vi "Get Meta Data.vi"(0 "Measurement Client Wrapper in":refnum<class "Measurement Client Wrapper.lvclass">, 11 "error in":errorcluster) -> (4 "Measurement Client Wrapper out":refnum<class "Measurement Client Wrapper.lvclass">, 15 "error out":errorcluster)   [LabVIEW 2020, in "Measurement Client Wrapper.lvclass"]
uses:
  Measurement Client Wrapper.lvclass
  Measurement Client Wrapper.lvclass/Measurement Client Wrapper.ctl
  Typedefs/Measurement Parameters.ctl
  Typedefs/Measurement Parameter Details.ctl
  Typedefs/Measurement DataType.ctl
  Measurement_lv_client/Measurement_lv_client Class/Measurement_lv_client.lvclass
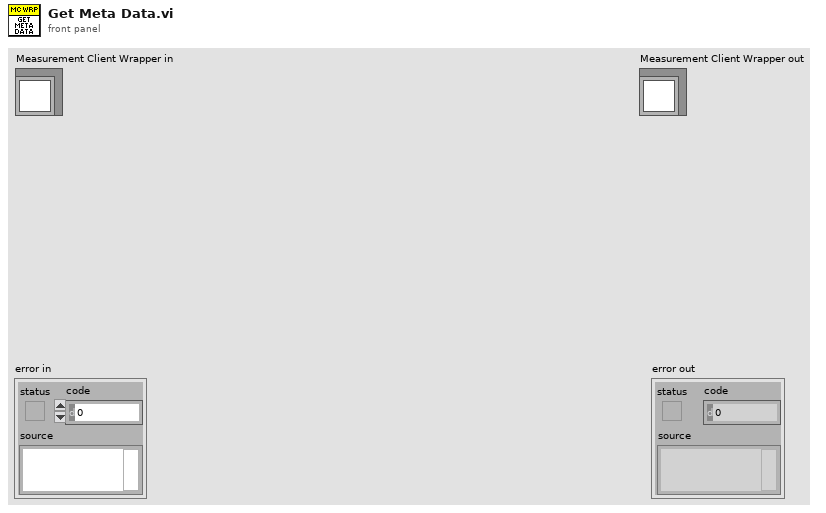
[diagram p1: front panel]
types:
  T1 = typedef "Measurement Client Wrapper.lvclass/Measurement Parameters.ctl" = cluster{"Configuration Parameters MessageType":string, "Configuration Parameter[]":T2[], "Output Parameters MessageType":string, "Output Parameter[]":T2[]}
  T2 = typedef "Measurement Client Wrapper.lvclass/Measurement Parameter Details.ctl" = cluster{"Name":string, "Parent":string, "ProtobufID":i32, "Measurement DataType":T3, "Array Dimension":i32}
  T3 = typedef "Measurement Client Wrapper.lvclass/Measurement DataType.ctl" = enum16{"UNSPECIFIED", "BOOL", "DOUBLE", "FLOAT", "INT32", "INT64", "STRING", "UINT32", "UINT64"}
  T4 = typedef "Measurement_lv_client.lvlib/Measurement_lv_client.lvclass/Measurement_v1_GetMetadataResponse_Data.ctl" = cluster{"measurement_details":T5, "measurement_parameters":T6, "user_interface_details":T9}
  T5 = typedef "Measurement_lv_client.lvlib/Measurement_lv_client.lvclass/Measurement_v1_MeasurementDetails_Data.ctl" = cluster{"display_name":string, "version":string, "measurement_type":string, "product_type":string}
  T6 = typedef "Measurement_lv_client.lvlib/Measurement_lv_client.lvclass/Measurement_v1_MeasurementParameters_Data.ctl" = cluster{"configuration_parameters_messagetype":string, "configuration_parameters":T7[], "output_parameters_messagetype":string, "output_parameters":T8[]}
  T7 = typedef "Measurement_lv_client.lvlib/Measurement_lv_client.lvclass/Measurement_v1_ConfigurationParameter_Data.ctl" = cluster{"protobuf_id":i32, "type":i32, "ArrayDimension":i32, "name":string, "parent":string}
  T8 = typedef "Measurement_lv_client.lvlib/Measurement_lv_client.lvclass/Measurement_v1_OutputParameter_Data.ctl" = cluster{"protobuf_id":i32, "type":i32, "ArrayDimension":i32, "name":string, "parent":string}
  T9 = typedef "Measurement_lv_client.lvlib/Measurement_lv_client.lvclass/Measurement_v1_UserInterfaceDetails_Data.ctl" = cluster{"configuration_ui_url":string}
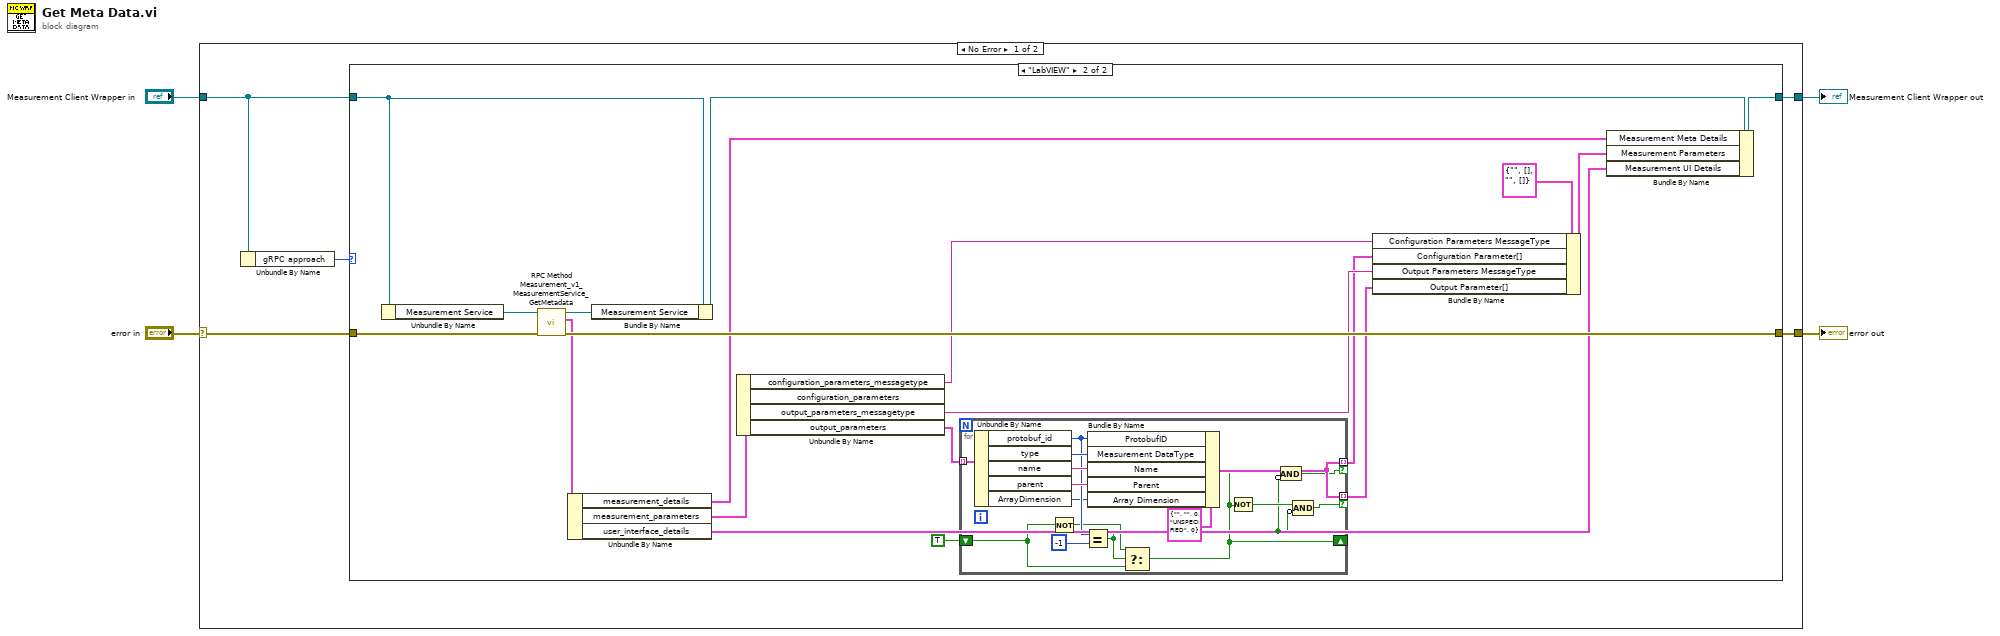
[diagram p0: block diagram]
diagram:
  n1 = case shown="No Error" "error in" {
    selector: "error in" -> [w9 w48]
    tunnel: [w7 w48] -> w3
    tunnel: [w8 w47] -> w1
    tunnel: "Measurement Client Wrapper in" -> [w6 w47]
    frame No Error {
      n2 = Unbundle By Name(w6) -> ("gRPC approach"=w5:enum16{".NET", "LabVIEW"})
      n3 = case shown="\"LabVIEW\"" w5 {
        tunnel: w9 -> [w11 w28]
        tunnel: [w10 w13] -> w8
        tunnel: [w11 w27] -> w7
        tunnel: w6 -> [w10 w30]
        frame ".NET", Default {
        }
        frame "LabVIEW" {
          n4 = Unbundle By Name(w30) -> ("Measurement Service"=w29:refnum<class "Measurement_lv_client.lvclass">)
          n5 = call "RPC Method Measurement_v1_MeasurementService_GetMetadata.vi"("error in (no error)"=w28, "gRPC Client in"=w29) -> ("error out"=w27:errorcluster, "Response Data"=w25:T4, "gRPC Client out"=w26:refnum<class "Measurement_lv_client.lvclass">)  [unwired: 7 in]
          n6 = Unbundle By Name(w25) -> ("measurement_details"=w16:T5, "measurement_parameters"=w24:T6, "user_interface_details"=w14:T9)
          n7 = Bundle By Name(cluster=w30, "Measurement Service"=w26) -> (w17:refnum<class "Measurement Client Wrapper.lvclass">)
          n8 = Unbundle By Name(w24) -> ("configuration_parameters_messagetype"=w20:string, "output_parameters_messagetype"=w21:string, "output_parameters"=w23:T8[])  [unwired: 1 out]
          n9 = for {
            tunnel: w23 -> [w46] mode=indexing
            tunnel: [w37] -> w12 mode=indexing if=w35
            shift-right: [w36] -> _
            shift-left: TRUE -> [w39]
            tunnel: [w37] -> w18 mode=indexing if=w32
            n10 = Unbundle By Name(w46) -> ("protobuf_id"=w41:i32, "type"=w45:i32, "name"=w44:string, "parent"=w43:string, "ArrayDimension"=w31:i32)
            n11 = Not(x=w39) -> (.not. x?=w38:bool)
            n12 = Equal?(x=w41, y=-1) -> (x = y?=w33:bool)
            n13 = Bundle By Name(cluster=T2 {"Name"="", "Parent"="", "ProtobufID"=0, "Measurement DataType"=enum."UNSPECIFIED", "Array Dimension"=0} ("Measurement Parameter Details"), "ProtobufID"=w41, "Measurement DataType"=w45, "Name"=w44, "Parent"=w43, "Array Dimension"=w31) -> (w37:T2)
            n14 = Select(t=w38, s=w33, f=w39) -> (s? t:f=w36:bool)
            n15 = Not(x=w36) -> (.not. x?=w34:bool)
            n16 = Compound Arithmetic op=AND(w36, invert w33) -> (w35:bool)
            n17 = Compound Arithmetic op=AND(w34, invert w33) -> (w32:bool)
          }
          n18 = Bundle By Name(cluster=T1 {"Configuration Parameters MessageType"="", "Configuration Parameter[]"=[], "Output Parameters MessageType"="", "Output Parameter[]"=[]} ("Measurement Parameters"), "Configuration Parameters MessageType"=w20, "Configuration Parameter[]"=w12, "Output Parameters MessageType"=w21, "Output Parameter[]"=w18) -> (w15:T1)
          n19 = Bundle By Name(cluster=w17, "Measurement Meta Details"=w16, "Measurement Parameters"=w15, "Measurement UI Details"=w14) -> (w13:refnum<class "Measurement Client Wrapper.lvclass">)
        }
      }
    }
    frame Error {
    }
  }
  "error out" <- w3
  "Measurement Client Wrapper out" <- w1
